vi "LVClass_CameraSet Get Parameter String Size.vi"(0 "CameraSet.lvclass":refnum<class "CameraSet.lvclass">, 5 "parameter name":string, 11 "error in (no error)":errorcluster) -> (4 "CameraSet.lvclass":refnum<class "CameraSet.lvclass">, 6 "size":i32, 15 "error out":errorcluster)   [LabVIEW 2020, in "CameraSet.lvclass"]
doc: "If parameter is a string to be selected among a finite set of strings, return\nthe size of this set. see Imop_CameraSet_GetParameterOption.\n\n<B>camera_setIn</B> : CameraSet object\n<B>camera_setOut</B> : CameraSet object\n<B>parameter_name</B> : Parameter name.\n<B>size</B> : Size of the list (count of strings expected in that parameter)."
uses:
  CameraSet.lvclass
  CameraSet.lvclass/CameraSet.ctl
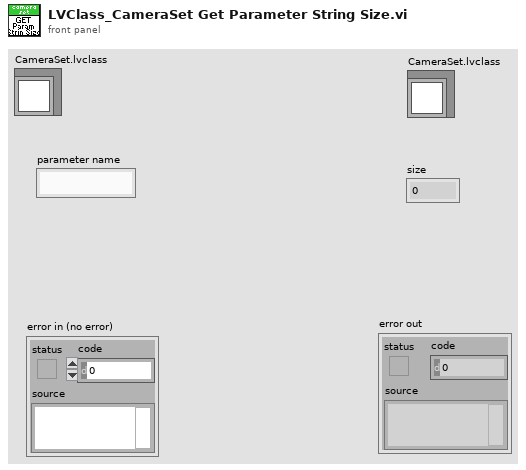
[diagram p1: front panel]
types:
  T1 = typedef "ClassID.ctl" = i64
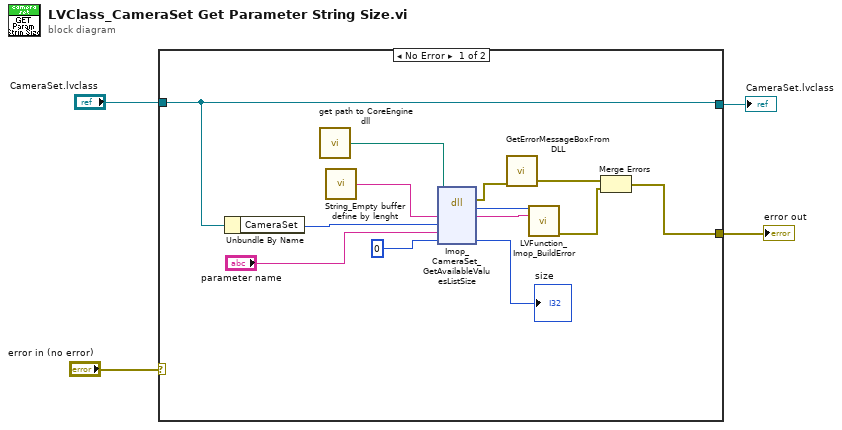
[diagram p0: block diagram]
diagram:
  n1 = case shown="No Error" "error in (no error)" {
    selector: "error in (no error)" -> [_ w18]
    tunnel: "CameraSet.lvclass" -> [w9 w19]
    tunnel: [w9 w19] -> w2
    tunnel: [w5 w18] -> w1
    frame No Error {
      n2 = Unbundle By Name(w9) -> ("CameraSet"=w8:T1)
      n3 = call "get path to CoreEngine dll.vi"() -> ("path to wavekit library"=w12:path)  [unwired: 14 in, 1 out]
      n4 = call "String_Empty buffer define by lenght.vi"() -> ("Empty buffer"=w15:string)  [unwired: 1 in]
      n5 = dll-call lib="D:/soft/HASO_v3/SVN_trunk/ImOpCoreEngine4_LV2011/DLLs/c_interface_vc100.dll" fn="Imop_CameraSet_GetAvailableValuesListSize"(path in=w12, "message"=w15, "objet"=w8, "parameter name"="parameter name", "size"=u32 0) -> (error out=w11:errorcluster, "return type"=w17:i32, "message"=w16:string, "size"=→"size":i32)  [unwired: 4 in, 1 out]
      n6 = call "GetErrorMessageBoxFromDLL.vi"("error IN"=w11) -> ("error OUT"=w7:errorcluster)  [unwired: 10 in]
      n7 = call "LVFunction_Imop_BuildError.vi"("code"=w17, "String to Prepend to source (\"\")"=w16) -> ("error out"=w6:errorcluster)  [unwired: 13 in]
      n8 = Merge Errors(w7, w6) -> (w5:errorcluster)
    }
    frame Error {
    }
  }
  "CameraSet.lvclass" <- w2
  "error out" <- w1
